vi "Get key value (Write JSON).vi"(0 "Single element name":string, 5 "previous\n level\n cluster":variant, 9 "Object name":string, 11 "error in (no error)":errorcluster) -> (4 "index out":i32, 6 "key":string, 8 "VArray":variant, 10 "value":string, 13 "Element Present?":bool, 14 "Array Present?":bool, 15 "error out":errorcluster)   [LabVIEW 2015]
uses:
  <vilib>/regexp/Match Regular Expression.xnode
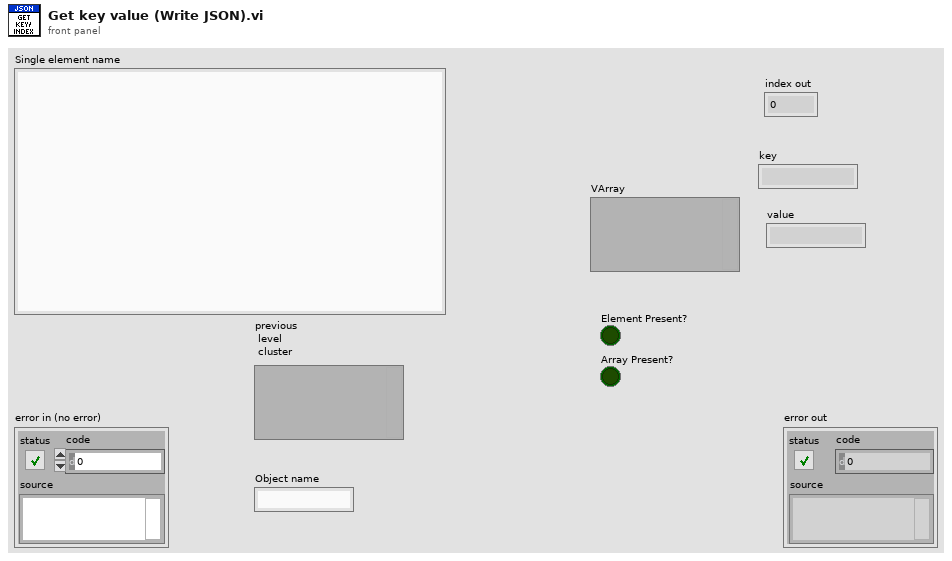
[diagram p1: front panel]
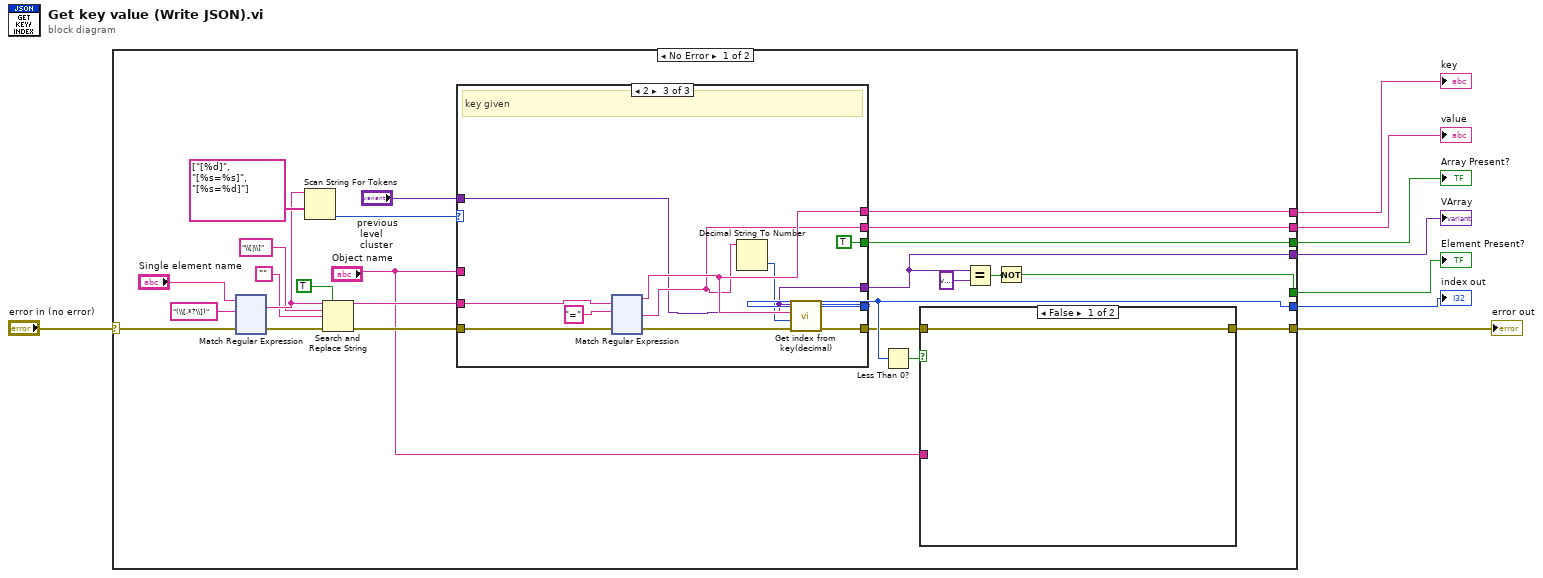
[diagram p0: block diagram]
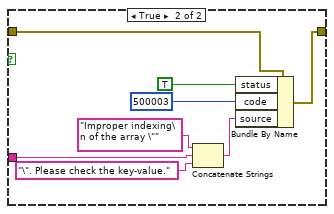
[diagram p2: hidden frame]
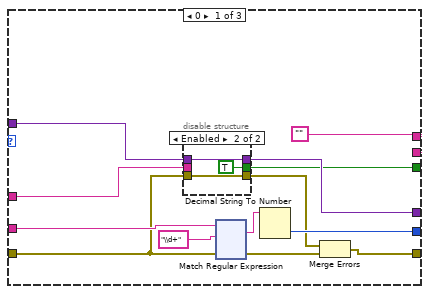
[diagram p3: hidden frame]
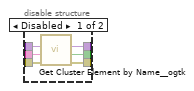
[diagram p4: hidden frame]
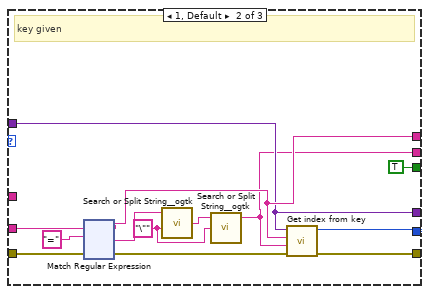
[diagram p5: hidden frame]
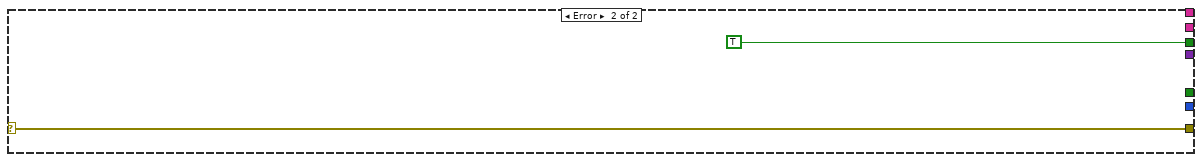
[diagram p6: hidden frame]
diagram:
  n1 = case shown="No Error" "error in (no error)" {
    selector: "error in (no error)" -> [w22 w546]
    tunnel: [w12 w546] -> w7
    tunnel: [w13 _] -> w6
    tunnel: [w21 _] -> w5
    tunnel: [w20 _] -> w4
    tunnel: [w18 TRUE ("found?")] -> w3
    tunnel: [w14 _] -> w2
    tunnel: [w15 _] -> w1
    frame No Error {
      n2 = xnode "Match Regular Expression"("input string"="Single element name", "regular expression"="(\\[.*?\\])", "error in"=w22) -> ("whole match"=w30:string, "error out"=w23:errorcluster)  [unwired: 3 in, 3 out]
      n3 = Scan String For Tokens(7:string[] ["[%d]", "[%s=%s]", "[%s=%d]"] ("operators (none)"), 9:w30) -> (0:w25:i32)  [unwired: 4 in, 3 out]
      n4 = Search and Replace String(replace all?=TRUE ("replace all? (F)"), input string=w30, search string="\\[|\\]", replace string="", error in=w23) -> (result string=w27:string, error out=w24:errorcluster)  [unwired: 3 in, 2 out]
      n5 = case shown="2" w25 {
        tunnel: w27 -> [w55 w191 w316]
        tunnel: w24 -> [w46 w190 w314]
        tunnel: [w52 w189 w313] -> w13
        tunnel: [w44 w188 w312] -> w11
        tunnel: [w51 w187 w311] -> w21
        tunnel: [w51 w179 w310] -> w20
        tunnel: [w48 w183 w308] -> w14
        tunnel: "Object name" -> [w49 _ _]
        tunnel: "previous\n level\n cluster" -> [w50 w183 w308]
        tunnel: [w47 TRUE ("found?") TRUE ("found?")] -> w18
        frame 0 {
          w51 = ""
          n6 = disable-structure shown="Enabled" {
            disable-tunnel: w50 -> [w61 w63]
            disable-tunnel: w49 -> [w60 _]
            disable-tunnel: [w59 w63] -> w48
            disable-tunnel: [w58 TRUE ("found?")] -> w47
            disable-tunnel: w46 -> [w57 w64]
            disable-tunnel: [w56 w64] -> w43
            frame Disabled {
              n7 = call <userlib>:"Get Cluster Element by Name__ogtk.vi"("error in (no error)"=w57, "Element Name"=w60, "Cluster"=w61) -> ("error out"=w56:errorcluster, "found?"=w58:bool, "VElement"=w59:variant)  [unwired: 6 in]
            }
            frame Enabled {
            }
          }
          n8 = xnode "Match Regular Expression"("input string"=w55, "regular expression"="\\d+", "error in"=w46) -> ("whole match"=w53:string, "error out"=w45:errorcluster)  [unwired: 3 in, 3 out]
          n9 = Decimal String To Number(string=w53) -> (number=w52:i32)  [unwired: 2 in, 1 out]
          n10 = Merge Errors(w43, w45) -> (w44:errorcluster)
        }
        frame 1, Default {
          w181 = "\"" ("search string/char (-)")
          # "key given"
          n11 = xnode "Match Regular Expression"("input string"=w191, "regular expression"="=", "error in"=w190) -> ("before match"=w187:string, "after match"=w180:string, "error out"=w185:errorcluster)  [unwired: 3 in, 2 out]
          n12 = call <userlib>:"Search or Split String__ogtk.vi"("search string/char (-)"=w181, "string"=w180) -> ("substring after match"=w182:string)  [unwired: 1 in, 2 out]
          n13 = call <userlib>:"Search or Split String__ogtk.vi"("search string/char (-)"=w181, "string"=w182) -> ("substring before match"=w179:string)  [unwired: 1 in, 2 out]
          n14 = call "Get index from key.vi"("error in (no error)"=w185, "value"=w179, "key"=w187, "VElement"=w183) -> ("error out"=w188:errorcluster, "indexOut"=w189:i32)  [unwired: 6 in]
        }
        frame 2 {
          # "key given"
          n15 = xnode "Match Regular Expression"("input string"=w316, "regular expression"="=", "error in"=w314) -> ("before match"=w311:string, "after match"=w310:string, "error out"=w307:errorcluster)  [unwired: 3 in, 2 out]
          n16 = Decimal String To Number(string=w310) -> (number=w309:i32)  [unwired: 2 in, 1 out]
          n17 = call "Get index from key(decimal).vi"("error in (no error)"=w307, "Value(decimal)"=w309, "key"=w311, "VElement"=w308) -> ("error out"=w312:errorcluster, "indexOut"=w313:i32)  [unwired: 6 in]
        }
      }
      n18 = Less Than 0?(x=w13) -> (x < 0?=w10:bool)
      n19 = case shown="False" w10 {
        tunnel: [w34 w39] -> w12
        tunnel: w11 -> [w34 w42]
        tunnel: "Object name" -> [_ w37]
        frame False {
        }
        frame True {
          n20 = Concatenate Strings("Improper indexing\n of the array \"" ("source"), w37, "\". Please check the key-value." ("string")) -> (w35:string)
          n21 = Bundle By Name(cluster=w42, "status"=TRUE, "code"=500003, "source"=w35) -> (w39:errorcluster)
        }
      }
      n22 = Equal?(x=w14, y=variant) -> (x = y?=w16:bool)
      n23 = Not(x=w16) -> (.not. x?=w15:bool)
    }
    frame Error {
    }
  }
  "error out" <- w7
  "index out" <- w6
  "key" <- w5
  "value" <- w4
  "Array Present?" <- w3
  "VArray" <- w2
  "Element Present?" <- w1
